vi "Apply Module Configuration Data.vi"(8 "Error In":errorcluster, 11 "Compiled.Settings":T1={"Name"="", "SLSC Name or IP Address"="", "Slot #"=0, "Configuration Data"={"Properties"={"Boolean Properties"=[], "Double Properties"=[], "I32 Properties"=[], "I64 Properties"=[], "String Properties"=[], "U32 Properties"=[], "U64 Properties"=[]}, "Commands"=[], "Reset Commands"=[], "Apply Values on Deployment"=TRUE, "Apply Reset on Undeployment"=TRUE, "Change Commands"=[]}, "SLSC Get/Read Properties"=[], "SLSC Set/Write Properties"=[], "SLSC Dynamic Commands"=[], "Support Modules"=[]}) -> (0 "Error Out":errorcluster, 2 "SLSC Module Name":refnum<k21>, 3 "Device Session":refnum<k21>)   [LabVIEW 2017]
uses:
  Shared/Compiled.Settings
  Shared/SLSC Static Settings.ctl
  SLSC CD API/SLSC CD Engine/SLSC Dynamic Channel.ctl
  SLSC CD API/SLSC CD Engine/SLSC Datatype.ctl
  <vilib>/SLSC/Initialize Session with Devices.vi
  SLSC EDS Engine.lvlib
  <vilib>/SLSC/SLSC.lvlib
  Shared/SLSC EDS Shared.lvlib
  SLSC CD API/SLSC CD Shared/SLSC CD Shared.lvlib
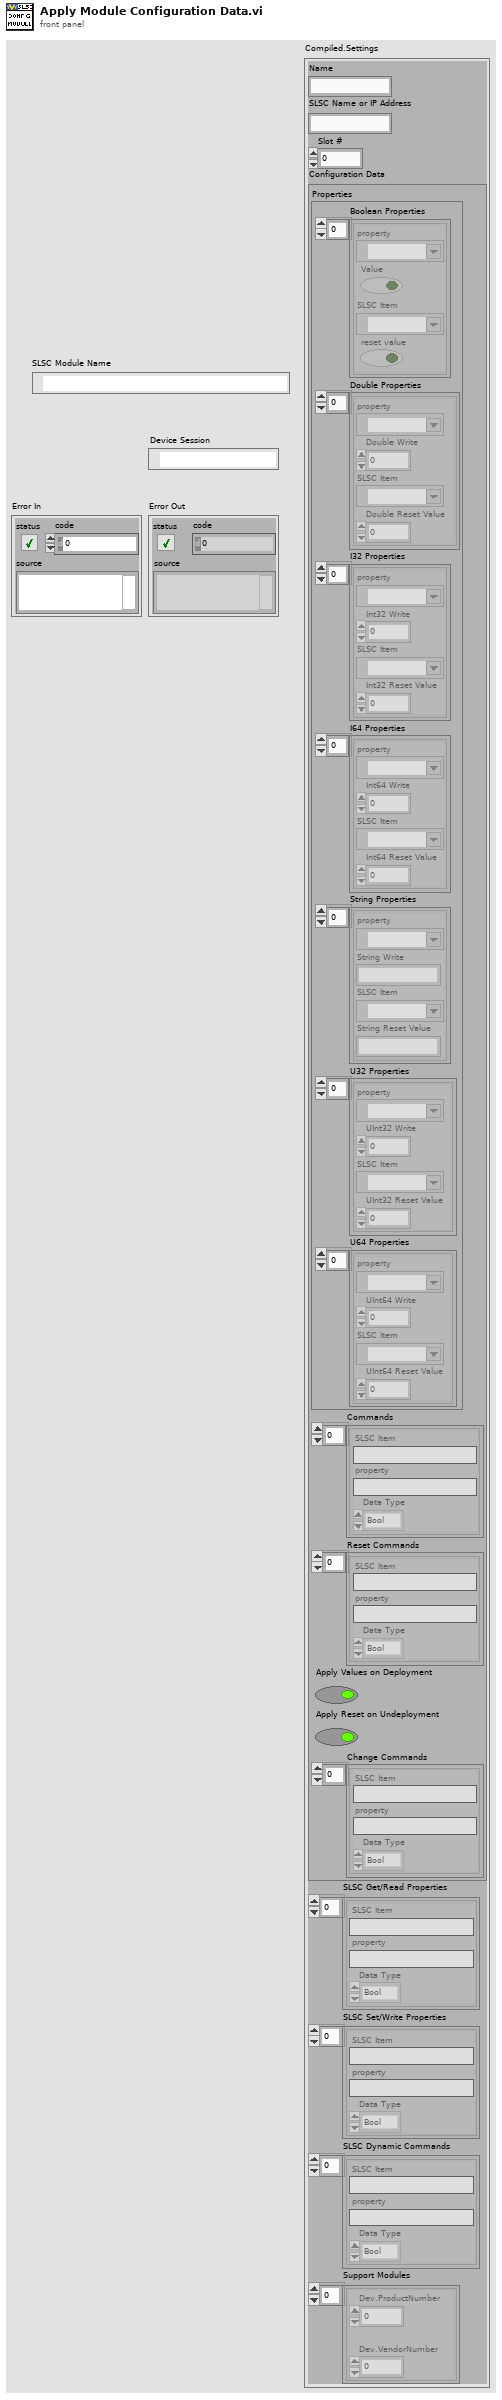
[diagram p1: front panel]
types:
  T1 = typedef "SLSC EDS Shared.lvlib/Compiled.Settings" = cluster{"Name":string, "SLSC Name or IP Address":string, "Slot #":i32, "Configuration Data":T2, "SLSC Get/Read Properties":T3[], "SLSC Set/Write Properties":T3[], "SLSC Dynamic Commands":T3[], "Support Modules":cluster{"Dev.ProductNumber":u32, "Dev.VendorNumber":u32}[]}
  T2 = typedef "SLSC EDS Shared.lvlib/SLSC Static Settings.ctl" = cluster{"Properties":cluster{"Boolean Properties":cluster{"property":refnum<k21>, "Value":bool, "SLSC Item":refnum<k21>, "reset value":bool}[], "Double Properties":cluster{"property":refnum<k21>, "Double Write":dbl, "SLSC Item":refnum<k21>, "Double Reset Value":dbl}[], "I32 Properties":cluster{"property":refnum<k21>, "Int32 Write":i32, "SLSC Item":refnum<k21>, "Int32 Reset Value":i32}[], "I64 Properties":cluster{"property":refnum<k21>, "Int64 Write":i64, "SLSC Item":refnum<k21>, "Int64 Reset Value":i64}[], "String Properties":cluster{"property":refnum<k21>, "String Write":string, "SLSC Item":refnum<k21>, "String Reset Value":string}[], "U32 Properties":cluster{"property":refnum<k21>, "UInt32 Write":u32, "SLSC Item":refnum<k21>, "UInt32 Reset Value":u32}[], "U64 Properties":cluster{"property":refnum<k21>, "UInt64 Write":u64, "SLSC Item":refnum<k21>, "UInt64 Reset Value":u64}[]}, "Commands":T3[], "Reset Commands":T3[], "Apply Values on Deployment":bool, "Apply Reset on Undeployment":bool, "Change Commands":T3[]}
  T3 = typedef "SLSC CD Shared.lvlib/SLSC Dynamic Channel.ctl" = cluster{"SLSC Item":string, "property":string, "Data Type":T4}
  T4 = typedef "SLSC CD Shared.lvlib/SLSC Datatype.ctl" = enum16{"Bool", "Double", "I32", "I64", "String", "U32", "U64"}
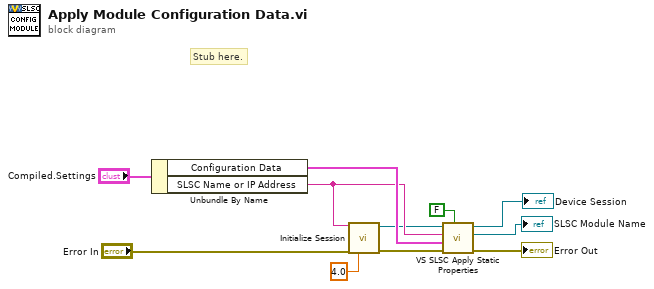
[diagram p0: block diagram]
diagram:
  # "Stub here."
  n1 = Unbundle By Name("Compiled.Settings") -> ("Configuration Data"=w10:T2, "SLSC Name or IP Address"=w8:string)
  n2 = call-poly <vilib>:"Initialize Session.vi"("devices"=w8, "error in (no error)"="Error In", "connect timeout (60 sec)"=4.0 ("connect timeout (10 sec)")) -> ("session out"=w3:refnum<k21>, "error out"=w4:errorcluster)  [unwired: 11 in]
  n3 = call "VS SLSC Apply Static Properties.vi"("Reset?"=FALSE, "error in (no error)"=w4, "Configuration Data"=w10, "SLSC Module Name in"=w8, "Refnum in"=w3) -> ("error out"=→"Error Out":errorcluster, "SLSC Module Name out"=→"SLSC Module Name":refnum<k21>, "Refnum out"=→"Device Session":refnum<k21>)  [unwired: 4 in]
